vi "SubVI_UpdateInput_002.vi"(6 "Encoder parameters":T1, 9 "Previous Input (in)":dbl, 10 "New info":i32) -> (3 "Input (out)":dbl)   [LabVIEW 2018]
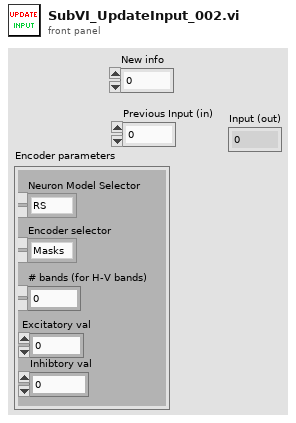
[diagram p1: front panel]
types:
  T1 = cluster{"Encoder selector":enum16{"Masks", "H-V bands", "Simple reading"}, "# bands (for H-V bands)":i32, "Excitatory val":dbl, "Inhibtory val":dbl, "Neuron Model Selector":enum16{"RS", "LTS", "RZ", "TC2", "TC1", "FS", "CH", "IB"}}
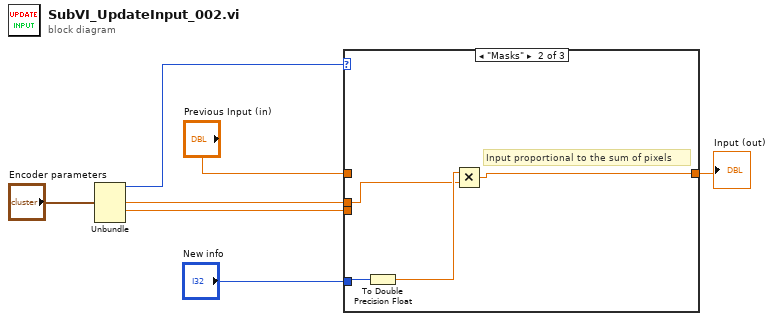
[diagram p0: block diagram]
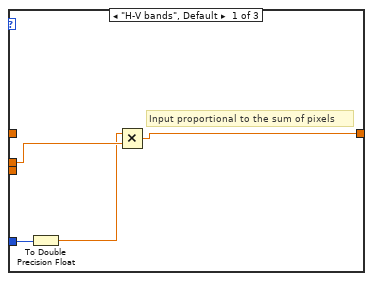
[diagram p2: hidden frame]
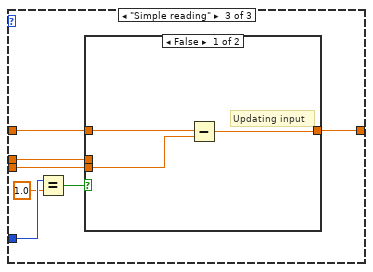
[diagram p3: hidden frame]
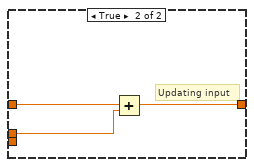
[diagram p4: hidden frame]
diagram:
  n1 = Unbundle("Encoder parameters") -> ("Encoder selector"=w2:enum16{"Masks", "H-V bands", "Simple reading"}, "Excitatory val"=w3:dbl, "Inhibtory val"=w4:dbl)  [unwired: 2 out]
  n2 = case shown="\"Masks\"" w2 {
    tunnel: w3 -> [w10 w14 w22]
    tunnel: [w11 w12 w21] -> w7
    tunnel: "Previous Input (in)" -> [_ _ w20]
    tunnel: w4 -> [_ _ w19]
    tunnel: "New info" -> [w9 w13 w17]
    frame "H-V bands", Default {
      # "Input proportional to the sum of pixels"
      n3 = To Double Precision Float(number=w9) -> (double precision float=w8:dbl)
      n4 = Multiply(x=w8, y=w10) -> (x*y=w11:dbl)
    }
    frame "Masks" {
      # "Input proportional to the sum of pixels"
      n5 = To Double Precision Float(number=w13) -> (double precision float=w15:dbl)
      n6 = Multiply(x=w15, y=w14) -> (x*y=w12:dbl)
    }
    frame "Simple reading" {
      n7 = Equal?(x=w17, y=1.0) -> (x = y?=w18:bool)
      n8 = case shown="False" w18 {
        tunnel: w20 -> [w25 w28]
        tunnel: [w24 w27] -> w21
        tunnel: w22 -> [_ w26]
        tunnel: w19 -> [w23 _]
        frame False {
          # "Updating input"
          n9 = Subtract(x=w25, y=w23) -> (x-y=w24:dbl)
        }
        frame True {
          # "Updating input"
          n10 = Add(x=w28, y=w26) -> (x+y=w27:dbl)
        }
      }
    }
  }
  "Input (out)" <- w7
